vi "RAM_DISK_USAGE (SubVI).vi"(11 "Refnum in":refnum<k21>="localhost" caption="Target (localhost)") -> (2 "Used Disk(%)":dbl, 3 "Used RAM(%)":dbl)   [LabVIEW 2022 SP3]
uses:
  <vilib>/nisyscfg/nisyscfg.lvlib
  <resource>/objmgr/nisysapi.rc
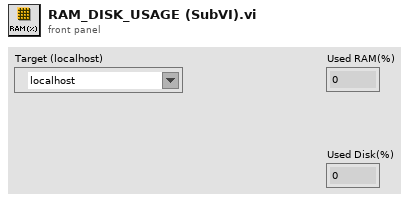
[diagram p1: front panel]
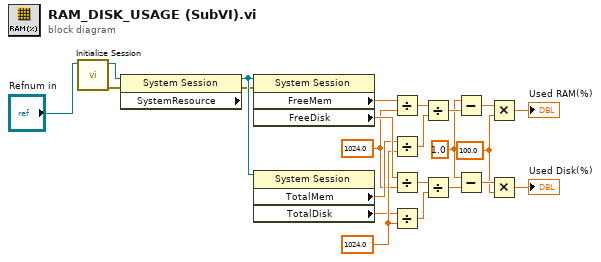
[diagram p0: block diagram]
diagram:
  w7 = 100.0 ("y")
  w6 = 1.0 ("x")
  w5 = 1024.0 ("y")
  w1 = 1024.0 ("y")
  n1 = call <vilib>:"Initialize Session.vi"("Target (localhost)"="Refnum in") -> ("error out"=w22:errorcluster, "Session out"=w21:refnum<k21>)  [unwired: 9 in]
  n2 = property class="System Session" props=["SystemResource"](reference=w21, error in=w22) -> (reference out=w23:refnum<k21>, error out=w2:errorcluster)  [unwired: 1 out]
  n3 = property class="System Session"(reference=w23, error in=w2) -> ("FreeMem"=w8:dbl, "FreeDisk"=w9:dbl)  [unwired: 2 out]
  n4 = property class="System Session"(reference=w23) -> ("TotalMem"=w3:dbl, "TotalDisk"=w4:dbl)  [unwired: 1 in, 2 out]
  n5 = Divide(x=w8, y=w1) -> (x/y=w10:dbl)
  n6 = Divide(x=w3, y=w5) -> (x/y=w11:dbl)
  n7 = Divide(x=w9, y=w1) -> (x/y=w13:dbl)
  n8 = Divide(x=w4, y=w5) -> (x/y=w14:dbl)
  n9 = Divide(x=w10, y=w11) -> (x/y=w12:dbl)
  n10 = Divide(x=w13, y=w14) -> (x/y=w15:dbl)
  n11 = Subtract(x=w6, y=w12) -> (x-y=w17:dbl)
  n12 = Subtract(x=w6, y=w15) -> (x-y=w16:dbl)
  n13 = Multiply(x=w17, y=w7) -> (x*y=→"Used RAM(%)":dbl)
  n14 = Multiply(x=w16, y=w7) -> (x*y=→"Used Disk(%)":dbl)
